vi "auto statelogger.vi"(8 "Rule name":string, 9 "Time":dbl format="%.2f", 10 "Plant State":T1=1 items=["OFF"], 11 "Datalog directory path":path) -> (0 "File Failure":bool)   [LabVIEW 2019]
uses:
  Plant state.ctl
  logic buffer cmd.ctl
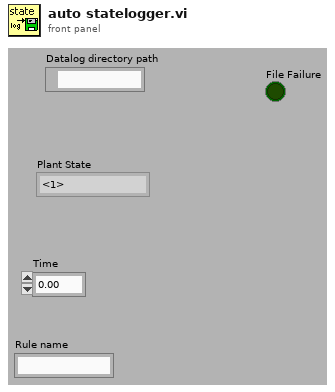
[diagram p1: front panel]
types:
  T1 = typedef "Plant state.ctl" = u16
  T2 = enum16{"open", "open or create", "create or replace", "create", "open (read only)"}
  T3 = typedef "logic buffer cmd.ctl" = enum16{"read", "write ouput settings", "write rules", "write setpoints", "write output descriptions", "write all", "calculate setpoints", "save", "open", "Load all setpoint code", "Load one setpoint code", "Configure one setpoint code"}
  T4 = typedef "rules.ctl" = T5[]
  T5 = typedef "State rules.ctl" = cluster{"state rules":T6[], "State name":string}
  T6 = typedef "rule.ctl" = cluster{"next state":u16, "conditions":T7[], "number of conditions":u8, "Rule name":string}
  T7 = typedef "condition.ctl" = cluster{"> or <":T8, "set point":i32, "sensors and variables":i32, "Data average interval":dbl}
  T8 = typedef "greater or less.ctl" = bool
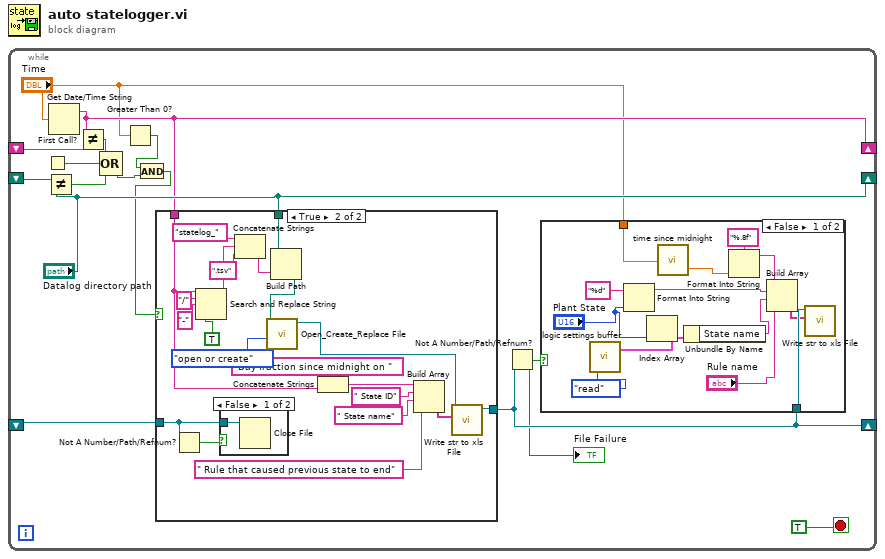
[diagram p0: block diagram]
diagram:
  n1 = while {
    shift-left: _ -> [w15]
    shift-right: ["Datalog directory path"] -> _
    shift-right: [w6] -> _
    shift-left: _ -> [w13]
    shift-right: [w8] -> _
    shift-left: _ -> [w7]
    stop <- TRUE stop-if-true
    n2 = First Call?() -> (First Call?: T/F=w11:bool)
    n3 = Not Equal?(x=w15, y="Datalog directory path") -> (x != y?=w10:bool)
    n4 = Get Date/Time String(seconds (now)="Time") -> (date string=w6:string)  [unwired: 2 in, 1 out]
    n5 = Not Equal?(x=w6, y=w13) -> (x != y?=w12:bool)
    n6 = Compound Arithmetic op=OR(w12, w11, w10) -> (w4:bool)
    n7 = Greater Than 0?(x="Time") -> (x > 0?=w2:bool)
    n8 = And(x=w2, y=w4) -> (x .and. y?=w3:bool)
    n9 = case shown="True" w3 {
      tunnel: w7 -> [w16 w22]
      tunnel: [w16 w37] -> w8
      tunnel: "Datalog directory path" -> [_ w33]
      tunnel: w6 -> [_ w23]
      frame False {
      }
      frame True {
        n10 = Not A Number/Path/Refnum?(number/path/refnum=w22) -> (NaN/Path/Refnum?=w21:bool)
        n11 = Search and Replace String(replace all?=TRUE ("replace all? (F)"), input string=w23, search string="/", replace string="-" ("replace string (\"\")")) -> (result string=w30:string)  [unwired: 4 in, 3 out]
        n12 = case shown="False" w21 {
          tunnel: w22 -> [w38 _]
          frame False {
            n13 = Close File(refnum=w38) -> ()  [unwired: 1 in, 2 out]
          }
          frame True {
          }
        }
        n14 = Concatenate Strings("statelog_" ("string"), w30, ".tsv" ("string")) -> (w29:string)
        n15 = Build Path(base path=w33, name or relative path=w29) -> (appended path=w28:path)
        n16 = call <vilib>:"Open_Create_Replace File.vi"("function (open:0)"=T2."open or create", "file path"=w28) -> ("refnum"=w26:refnum<file>)  [unwired: 6 in, 3 out]
        n17 = Concatenate Strings("Day fraction since midnight on " ("Substring"), w23) -> (w25:string)
        n18 = Build Array(w25, " State ID" ("Substring"), " State name" ("Substring"), " Rule that caused previous state to end" ("Substring")) -> (w19:string[])
        n19 = call "Write str to xls File.vi"("1D data"=w19, "refnum"=w26) -> ("dup refnum"=w37:refnum<file>)  [unwired: 8 in, 1 out]
      }
    }
    n20 = Not A Number/Path/Refnum?(number/path/refnum=w8) -> (NaN/Path/Refnum?=w5:bool)
    "File Failure" <- w5
    n21 = case shown="False" w5 {
      tunnel: w8 -> [w52 _]
      tunnel: "Time" -> [w46 _]
      frame False {
        n22 = call "logic settings buffer.vi"("command"=logic_buffer_cmd."read") -> ("Rules out"=w43:T4)  [unwired: 11 in, 7 out]
        n23 = Format Into String(format string="%d", "Plant State") -> (resulting string=w48:string)  [unwired: 2 in, 1 out]
        n24 = Index Array(array=w43, index="Plant State") -> (element=w41:T5)
        n25 = call "time since midnight.vi"("seconds since 1Jan1904"=w46) -> ("Days"=w51:dbl)  [unwired: 1 out]
        n26 = Unbundle By Name(w41) -> ("State name"=w40:string)
        n27 = Format Into String(format string="%.8f" ("format (%.3f)"), w51) -> (resulting string=w47:string)  [unwired: 2 in, 1 out]
        n28 = Build Array(w47, w48, w40, "Rule name") -> (w45:string[])
        n29 = call "Write str to xls File.vi"("1D data"=w45, "refnum"=w52) -> ()  [unwired: 8 in, 2 out]
      }
      frame True {
      }
    }
  }
